vi "Encoder and Pockels task.vi"(8 "error in (no error)":errorcluster, 11 "Setup/Logging queue element":T2={"Imaging Protocol"=enum."Live Imaging", "Number of Trials"=0, "Frame Size"=512, "# Averaged frames"=0, "Dwell time (us)"=0.0, "Index of Z-plane"=0, "Timelapse?"=FALSE, "Logging process is active"=FALSE, "Speed logging enabled"=FALSE, "tdms file ref"=refnum, "path"=path "", "Trial Number"=0, "Expected # points acquired"=FALSE, "Manually stopped"=FALSE, "Ch0 data"=[], "Ch1 data"=[], "Last trial"=FALSE, "Points acquired"={"Ch0 last trial"=0, "Ch1 last trial"=0, "All trials"=0}} {"Frame Size" items=["100X100"=100, "128X128"=128, "200X200"=200, "256X256"=256, "512X512"=512, "1024x1024"=1024, "2048x2048"=2048]; "Dwell time (us)" format="%#.6g"}) -> (0 "error out":errorcluster)   [LabVIEW 2013]
uses:
  Typedefs/Logging queue element.ctl
  Typedefs/Imaging Protocols enum.ctl
  Typedefs/Frame Size.ctl
  Typedefs/Acquired points count.ctl
  Typedefs/Triggered tasks cluster.ctl
  Globals/gl_Triggering globals.vi
panel:
  out "Info":T1 {"Sampling period (us)" format="%#_6f"; "Data lenght (ms)" format="%#_6f"}
  out "# of DO points":i32
  out "Digital Waveform Graph":digitaldata(graph)
  out "Waveform Graph":dbl[](graph)
  out "# of AO points":i32
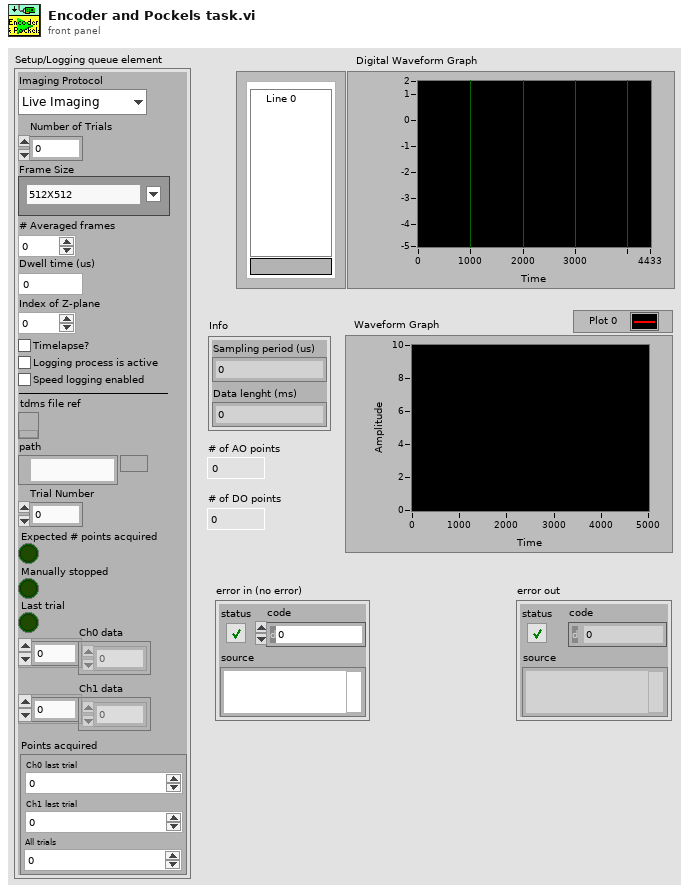
[diagram p1: front panel]
types:
  T1 = cluster{"Sampling period (us)":dbl, "Data lenght (ms)":dbl}
  T2 = typedef "Logging queue element.ctl" = cluster{"Imaging Protocol":T3, "Number of Trials":u16, "Frame Size":T4, "# Averaged frames":u16, "Dwell time (us)":dbl, "Index of Z-plane":i32, "Timelapse?":bool, "Logging process is active":bool, "Speed logging enabled":bool, "tdms file ref":refnum<k34>, "path":path, "Trial Number":i32, "Expected # points acquired":bool, "Manually stopped":bool, "Ch0 data":u32[], "Ch1 data":u32[], "Last trial":bool, "Points acquired":T5}
  T3 = typedef "Imaging Protocols enum.ctl" = enum16{"AOL Z-Stack", "Motor Z Stack", "Functional Acquisition", "Single Plane Acquisition", "Volume Acquisition", "Live Imaging", "Live Plane Imaging", "Live Volume Imaging"}
  T4 = typedef "Frame Size.ctl" = u16
  T5 = typedef "Acquired points count.ctl" = cluster{"Ch0 last trial":u64, "Ch1 last trial":u64, "All trials":u64}
  T6 = typedef "Triggered tasks cluster.ctl" = cluster{"DO task-Encoder trigger":refnum<k21>, "AO Task-Pockels modulation":refnum<k21>, "Counter Clock Task":refnum<k21>}
  T7 = cluster{"Sampling period (us)":dbl, "Data length (ms)":dbl}
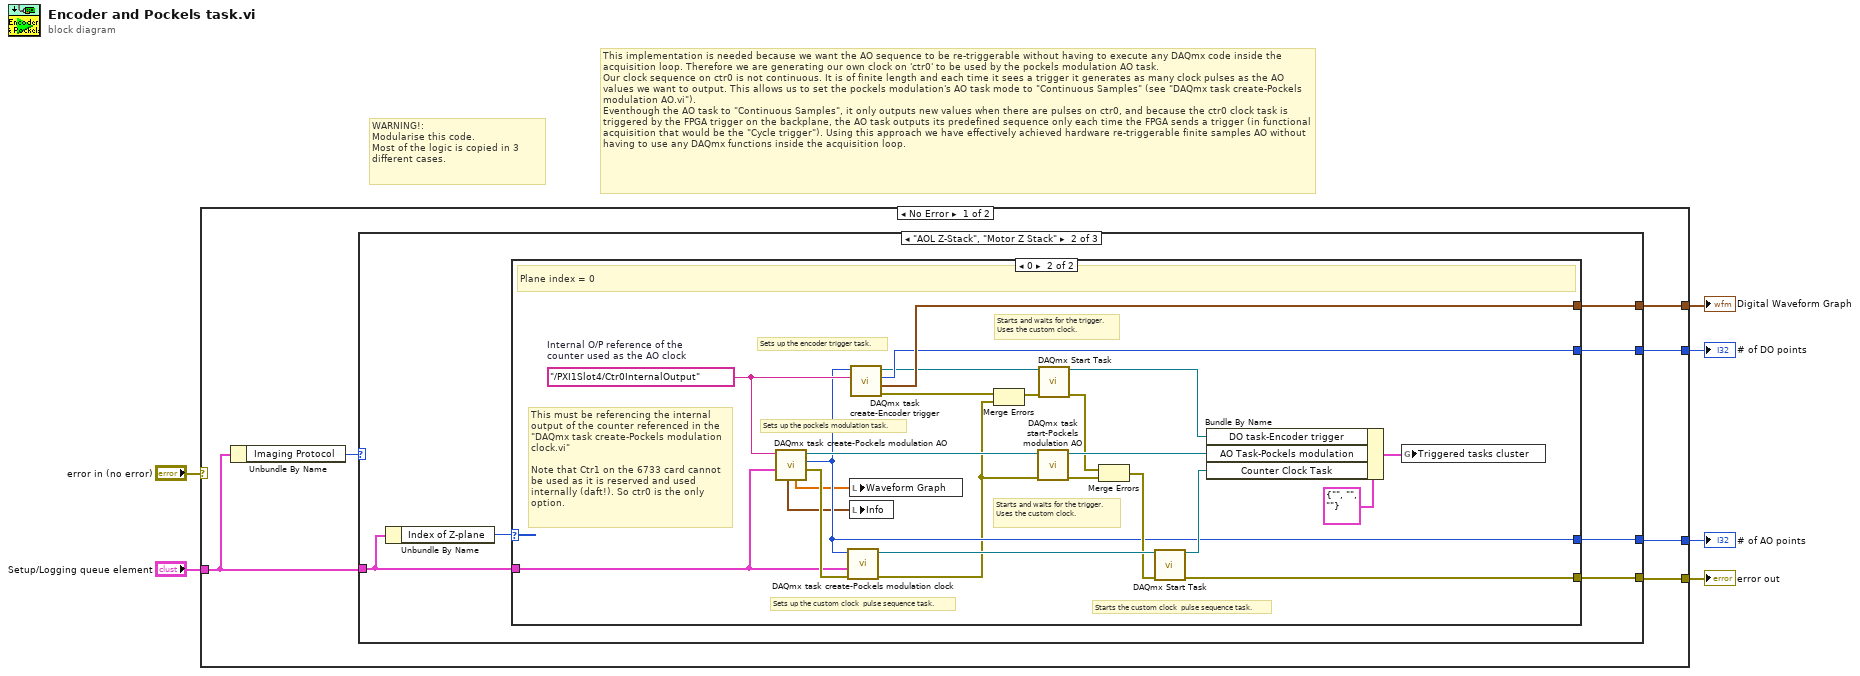
[diagram p0: block diagram]
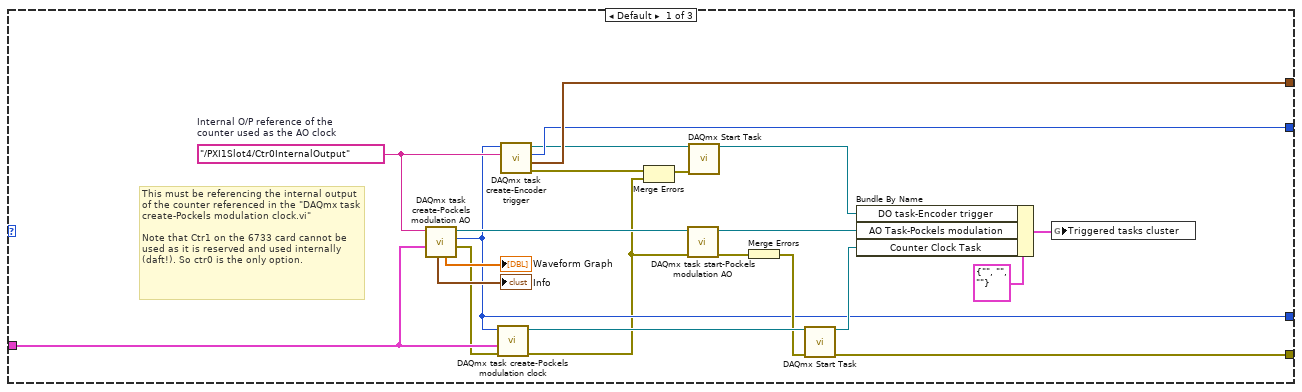
[diagram p2: hidden frame]
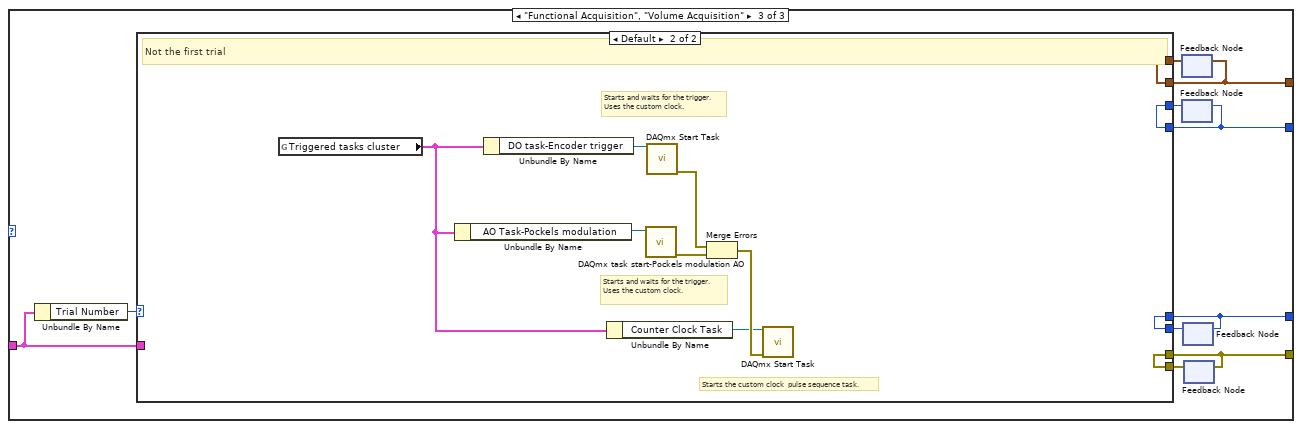
[diagram p4: hidden frame]
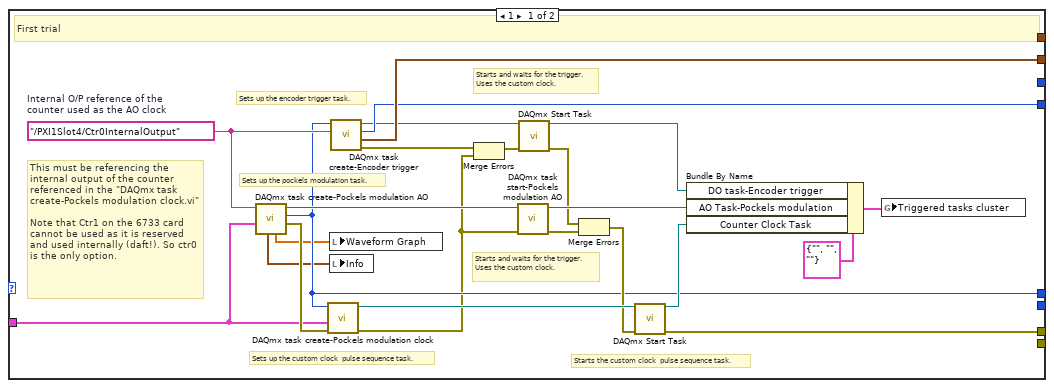
[diagram p5: hidden frame]
diagram:
  # "WARNING!:\nModularise this code.\nMost of the logic is copied in 3 different cases."
  # "This implementation is needed because we want the AO sequence to be re-triggerable without having to execute any DAQmx code inside the acquisition loop. Therefore we are generating our own clock on 'ctr0' to be used by the pockels modulation AO task.\nOur clock sequence on ctr0 is not continuous. It is of finite length and each time it sees a trigger it generates as many clock pulses as the AO values we want to output. This allows us to set the pockels modulation's AO task mode to \"Continuous Samples\" (see \"DAQmx task create-Pockels modulation AO.vi\").\nEventhough the AO task to \"Continuous Samples\", it only outputs new values when there are pulses on ctr0, and because the ctr0 clock task is triggered by the FPGA trigger on the backplane, the AO task outputs its predefined sequence only each time the FPGA sends a trigger (in functional acquisition that would be the \"Cycle trigger\"). Using this approach we have effectively achieved hardware re-triggerable finite samples AO without having to use any DAQmx functions inside the acquisition loop."
  n1 = case shown="No Error" "error in (no error)" {
    selector: "error in (no error)" -> [_ w108]
    tunnel: [w12 w108] -> w5
    tunnel: [w9 _] -> w4
    tunnel: [w11 _] -> w3
    tunnel: "Setup/Logging queue element" -> [w8 _]
    tunnel: [w10 _] -> w2
    frame No Error {
      n2 = Unbundle By Name(w8) -> ("Imaging Protocol"=w7:T3)
      n3 = case shown="\"AOL Z-Stack\", \"Motor Z Stack\"" w7 {
        tunnel: [w31 w40 w69] -> w12
        tunnel: [w28 w39 w71] -> w11
        tunnel: [w27 w38 w67] -> w10
        tunnel: w8 -> [w21 w36 w73]
        tunnel: [w16 w37 w68] -> w9
        frame Default {
          w20 = tag "/PXI1Slot4/Ctr0InternalOutput"  # Internal O/P reference of the  counter used as the AO clock
          # "This must be referencing the internal output of the counter referenced in the \"DAQmx task create-Pockels modulation clock.vi\"\n\nNote that Ctr1 on the 6733 card cannot be used as it is reserved and used internally (daft!). So ctr0 is the only option."
          n4 = call "DAQmx task create-Pockels modulation AO.vi"("Setup/Logging queue element"=w21, "Internal O/P reference of the \ncounter used as the AO clock"=w20) -> ("error out"=w18:errorcluster, "Data length (points)"=w16:i32, "Pockels modulation AO task"=w23:refnum<k21>, "Info"=→"Info":T7, "Pockels modulation data out"=→"Waveform Graph":dbl[])  [unwired: 5 in]
          n5 = call "DAQmx task create-Pockels modulation clock.vi"("error in"=w18, "Setup/Logging queue element"=w21, "Data length"=w16) -> ("error out"=w15:errorcluster, "Refnum out"=w25:refnum<k21>)  [unwired: 7 in]
          n6 = call "DAQmx task create-Encoder trigger.vi"("Internal O/P reference of the \ncounter used as the AO clock"=w20, "Data length"=w16) -> ("error out"=w14:errorcluster, "Encoder trigger DO sequence"=w28:digitaldata, "# points in output waveform"=w27:i32, "Refnum out"=w13:refnum<k21>)  [unwired: 6 in]
          n7 = Merge Errors(w14, w15) -> (w17:errorcluster)
          n8 = call "DAQmx task start-Pockels modulation AO.vi"("error in (no error)"=w15, "Pockels modulation AO task in"=w23) -> ("error out"=w26:errorcluster, "Pockels modulation AO task out"=w29:refnum<k21>)  [unwired: 8 in]
          n9 = call <vilib>:"DAQmx Start Task.vi"("task/channels in"=w13, "error in"=w17) -> ("task out"=w30:refnum<k21>)  [unwired: 12 in, 1 out]
          n10 = Merge Errors(w26) -> (w24:errorcluster)
          n11 = call <vilib>:"DAQmx Start Task.vi"("task/channels in"=w25, "error in"=w24) -> ("task out"=w32:refnum<k21>, "error out"=w31:errorcluster)  [unwired: 12 in]
          n12 = Bundle By Name(cluster=T6 {"DO task-Encoder trigger"="", "AO Task-Pockels modulation"="", "Counter Clock Task"=""}, "DO task-Encoder trigger"=w30, "AO Task-Pockels modulation"=w29, "Counter Clock Task"=w32) -> (w34:T6)
          n13 = global write "gl_Triggering globals.vi" "Triggered tasks cluster"(w34) -> ()
        }
        frame "AOL Z-Stack", "Motor Z Stack" {
          n14 = Unbundle By Name(w36) -> ("Index of Z-plane"=w35:i32)
          n15 = case shown="0" w35 {
            tunnel: [_ w60] -> w40
            tunnel: [_ w57] -> w39
            tunnel: [_ w56] -> w38
            tunnel: [_ w48] -> w37
            tunnel: w36 -> [_ w44]
            frame Default {
              # "Plane index is other than zero"
            }
            frame 0 {
              w51 = tag "/PXI1Slot4/Ctr0InternalOutput"  # Internal O/P reference of the  counter used as the AO clock
              # "Sets up the pockels modulation task."
              # "Sets up the encoder trigger task."
              # "Sets up the custom clock  pulse sequence task."
              # "Starts the custom clock  pulse sequence task."
              # "Starts and waits for the trigger.\nUses the custom clock."
              # "Starts and waits for the trigger.\nUses the custom clock."
              # "This must be referencing the internal output of the counter referenced in the \"DAQmx task create-Pockels modulation clock.vi\"\n\nNote that Ctr1 on the 6733 card cannot be used as it is reserved and used internally (daft!). So ctr0 is the only option."
              # "Plane index = 0"
              n16 = call "DAQmx task create-Pockels modulation AO.vi"("Setup/Logging queue element"=w44, "Internal O/P reference of the \ncounter used as the AO clock"=w51) -> ("error out"=w50:errorcluster, "Data length (points)"=w48:i32, "Pockels modulation AO task"=w52:refnum<k21>, "Info"=w43:T7, "Pockels modulation data out"=w42:dbl[])  [unwired: 5 in]
              n17 = call "DAQmx task create-Pockels modulation clock.vi"("error in"=w50, "Setup/Logging queue element"=w44, "Data length"=w48) -> ("error out"=w47:errorcluster, "Refnum out"=w54:refnum<k21>)  [unwired: 7 in]
              n18 = local write "Waveform Graph"(w42) -> ()
              n19 = local write "Info"(w43) -> ()
              n20 = call "DAQmx task create-Encoder trigger.vi"("Internal O/P reference of the \ncounter used as the AO clock"=w51, "Data length"=w48) -> ("error out"=w46:errorcluster, "Encoder trigger DO sequence"=w57:digitaldata, "# points in output waveform"=w56:i32, "Refnum out"=w45:refnum<k21>)  [unwired: 6 in]
              n21 = Merge Errors(w46, w47) -> (w49:errorcluster)
              n22 = call "DAQmx task start-Pockels modulation AO.vi"("error in (no error)"=w47, "Pockels modulation AO task in"=w52) -> ("error out"=w55:errorcluster, "Pockels modulation AO task out"=w58:refnum<k21>)  [unwired: 8 in]
              n23 = call <vilib>:"DAQmx Start Task.vi"("task/channels in"=w45, "error in"=w49) -> ("task out"=w59:refnum<k21>, "error out"=w41:errorcluster)  [unwired: 12 in]
              n24 = Merge Errors(w41, w55) -> (w53:errorcluster)
              n25 = call <vilib>:"DAQmx Start Task.vi"("task/channels in"=w54, "error in"=w53) -> ("task out"=w61:refnum<k21>, "error out"=w60:errorcluster)  [unwired: 12 in]
              n26 = Bundle By Name(cluster=T6 {"DO task-Encoder trigger"="", "AO Task-Pockels modulation"="", "Counter Clock Task"=""}, "DO task-Encoder trigger"=w59, "AO Task-Pockels modulation"=w58, "Counter Clock Task"=w61) -> (w63:T6)
              n27 = global write "gl_Triggering globals.vi" "Triggered tasks cluster"(w63) -> ()
            }
          }
        }
        frame "Functional Acquisition", "Volume Acquisition" {
          n28 = Unbundle By Name(w73) -> ("Trial Number"=w72:i32)
          n29 = feedback #1() -> (w70:digitaldata)  [unwired: 1 in]
          n30 = feedback #2() -> (w66:i32)  [unwired: 1 in]
          n31 = feedback #3() -> (w65:i32)  [unwired: 1 in]
          n32 = feedback #4() -> (w64:errorcluster)  [unwired: 1 in]
          n33 = case shown="Default" w72 {
            tunnel: [w93 w101] -> w69
            tunnel: [w90 w104] -> w71
            tunnel: [w89 w103] -> w67
            tunnel: [w81 w102] -> w68
            tunnel: w73 -> [w77 _]
            tunnel: w70 -> [_ w104]
            tunnel: w66 -> [_ w103]
            tunnel: w65 -> [_ w102]
            tunnel: w64 -> [_ w101]
            frame 1 {
              w84 = tag "/PXI1Slot4/Ctr0InternalOutput"  # Internal O/P reference of the  counter used as the AO clock
              # "Sets up the pockels modulation task."
              # "Sets up the encoder trigger task."
              # "Sets up the custom clock  pulse sequence task."
              # "Starts the custom clock  pulse sequence task."
              # "Starts and waits for the trigger.\nUses the custom clock."
              # "Starts and waits for the trigger.\nUses the custom clock."
              # "This must be referencing the internal output of the counter referenced in the \"DAQmx task create-Pockels modulation clock.vi\"\n\nNote that Ctr1 on the 6733 card cannot be used as it is reserved and used internally (daft!). So ctr0 is the only option."
              # "First trial"
              n34 = call "DAQmx task create-Pockels modulation AO.vi"("Setup/Logging queue element"=w77, "Internal O/P reference of the \ncounter used as the AO clock"=w84) -> ("error out"=w83:errorcluster, "Data length (points)"=w81:i32, "Pockels modulation AO task"=w85:refnum<k21>, "Info"=w76:T7, "Pockels modulation data out"=w75:dbl[])  [unwired: 5 in]
              n35 = call "DAQmx task create-Pockels modulation clock.vi"("error in"=w83, "Setup/Logging queue element"=w77, "Data length"=w81) -> ("error out"=w80:errorcluster, "Refnum out"=w87:refnum<k21>)  [unwired: 7 in]
              n36 = local write "Waveform Graph"(w75) -> ()
              n37 = local write "Info"(w76) -> ()
              n38 = call "DAQmx task create-Encoder trigger.vi"("Internal O/P reference of the \ncounter used as the AO clock"=w84, "Data length"=w81) -> ("error out"=w79:errorcluster, "Encoder trigger DO sequence"=w90:digitaldata, "# points in output waveform"=w89:i32, "Refnum out"=w78:refnum<k21>)  [unwired: 6 in]
              n39 = Merge Errors(w79, w80) -> (w82:errorcluster)
              n40 = call "DAQmx task start-Pockels modulation AO.vi"("error in (no error)"=w80, "Pockels modulation AO task in"=w85) -> ("error out"=w88:errorcluster, "Pockels modulation AO task out"=w91:refnum<k21>)  [unwired: 8 in]
              n41 = call <vilib>:"DAQmx Start Task.vi"("task/channels in"=w78, "error in"=w82) -> ("task out"=w92:refnum<k21>, "error out"=w74:errorcluster)  [unwired: 12 in]
              n42 = Merge Errors(w74, w88) -> (w86:errorcluster)
              n43 = call <vilib>:"DAQmx Start Task.vi"("task/channels in"=w87, "error in"=w86) -> ("task out"=w94:refnum<k21>, "error out"=w93:errorcluster)  [unwired: 12 in]
              n44 = Bundle By Name(cluster=T6 {"DO task-Encoder trigger"="", "AO Task-Pockels modulation"="", "Counter Clock Task"=""}, "DO task-Encoder trigger"=w92, "AO Task-Pockels modulation"=w91, "Counter Clock Task"=w94) -> (w96:T6)
              n45 = global write "gl_Triggering globals.vi" "Triggered tasks cluster"(w96) -> ()
            }
            frame Default {
              # "Starts the custom clock  pulse sequence task."
              # "Starts and waits for the trigger.\nUses the custom clock."
              # "Starts and waits for the trigger.\nUses the custom clock."
              # "Not the first trial"
              n46 = global read "gl_Triggering globals.vi" "Triggered tasks cluster"() -> (w97:T6)
              n47 = Unbundle By Name(w97) -> ("AO Task-Pockels modulation"=w99:refnum<k21>)
              n48 = Unbundle By Name(w97) -> ("DO task-Encoder trigger"=w100:refnum<k21>)
              n49 = Unbundle By Name(w97) -> ("Counter Clock Task"=w98:refnum<k21>)
              n50 = call "DAQmx task start-Pockels modulation AO.vi"("Pockels modulation AO task in"=w99) -> ("error out"=w107:errorcluster)  [unwired: 9 in, 1 out]
              n51 = call <vilib>:"DAQmx Start Task.vi"("task/channels in"=w100) -> ("error out"=w105:errorcluster)  [unwired: 13 in, 1 out]
              n52 = Merge Errors(w105, w107) -> (w106:errorcluster)
              n53 = call <vilib>:"DAQmx Start Task.vi"("task/channels in"=w98, "error in"=w106) -> ()  [unwired: 12 in, 2 out]
            }
          }
          n54 = feedback-in #1(w71) -> ()
          n55 = feedback-in #2(w67) -> ()
          n56 = feedback-in #3(w68) -> ()
          n57 = feedback-in #4(w69) -> ()
        }
      }
    }
    frame Error {
    }
  }
  "error out" <- w5
  "# of AO points" <- w4
  "Digital Waveform Graph" <- w3
  "# of DO points" <- w2
